vi "RADAR (NI 5791 FPGA).vi"() -> ()   [LabVIEW 2017]
uses:
  <instrlib>/_niInstr/Register Bus/v1/FPGA/Public/Read Cmd Data.ctl
  <instrlib>/_niInstr/DSP/v1/Shared/Public/IQ Gain.ctl
  <instrlib>/_niInstr/DSP/v1/Shared/Public/IQ Impairments.ctl
  <vilib>/Platform/TimedLoop/XDataNode/timing_clust.ctl
  <vilib>/Platform/TimedLoop/XDataNode/nitl_modes.ctl
  <vilib>/Platform/TimedLoop/XDataNode/wakeup.ctl
  <instrlib>/_niInstr/DSP/v1/Shared/Public/IQ Data.ctl
  <instrlib>/ni579x/Synchronization/v2/FPGA/Implementation/Create 5791.vi
  <vilib>/rvi/Emulation/niFpgaSctlEmulationGetInTimedLoop.vi
  <vilib>/rvi/Emulation/niFpgaEmulationReportErrorSimple.vi
  <vilib>/rvi/Emulation/niFpgaGetClockAttributes.vi
  <vilib>/rvi/Emulation/niFpgaCriticalErrorInLSC.vi
  <vilib>/rvi/eio/common/nirviEmuTemplateMethod_errors.vi
  <instrlib>/_niInstr/Register Bus/v1/FPGA/Private/Mux/Read Completion Mux (3 inputs).vi
  <vilib>/rvi/Emulation/niFpgaProcessEmulError.vi
  <instrlib>/_niInstr/DSP/v1/FPGA/Public/Sub VIs/Data Conversion/I16 to IQ - 1 spc - S18.1.vi
  <instrlib>/_niInstr/DSP/v1/FPGA/Public/Sub VIs/Data Conversion/IQ to U32 - 1 spc - S18.1.vi
  <instrlib>/_niInstr/Basic Elements/v1/FPGA/Private/Count Up U64.vi
  <instrlib>/_niInstr/DSP/v1/FPGA/Public/Sub VIs/Data Conversion/U32 to IQ - 1 spc - S18.1.vi
  <instrlib>/_niInstr/DSP/v1/FPGA/Public/Sub VIs/Data Conversion/IQ to I16 - 1 spc - S18.1.vi
  <vilib>/rvi/interface/RandomDataEmulation/niFpgaRandomDataHandleErrors.vi
  <vilib>/rvi/DataTransferAndStorage/Container/Common/niFpgaContainerExecOnDevCompGetState.vi
  <vilib>/rvi/Emulation/niFpgaEmulationIsFPGAContextNoSignature.vi
  <vilib>/rvi/errors/niFpgaSetErrorForExecOnDevCompSimple.vi
  <vilib>/rvi/eio/common/nirviEmuReportErrorAndStop.vi
  <vilib>/rvi/DataTransferAndStorage/Container/Common/niFpgaContainerGetUniqueNameForEmu.vi
  <vilib>/rvi/FIFO/Fifo_Resource/nirvififoEmulationSetSize.vi
  <vilib>/rvi/FIFO/Fifo_Resource/nirviFifoEmulationQueueMgr.vi
  <instcachedir>/0/nirviFifoEmulationQueueMgr_E5CAEC123FF24DC58D834DCA3CDAA9B5.lvgen/nirviFifoEmulationQueueMgr_E5CAEC123FF24DC58D834DCA3CDAA9B5_000.vi
  <vilib>/rvi/FIFO/Fifo_Resource/nirvififoEmulationDetermineInputValidOut.vi
  <vilib>/rvi/FIFO/Fifo_Resource/nirvififoEmulationCreateLock.vi
  <vilib>/rvi/FIFO/Fifo_Resource/nirvififoEmulationObtainLock.vi
  <vilib>/rvi/FIFO/Fifo_Resource/nirvififoEmulationReleaseLock.vi
  <vilib>/rvi/occurrence/nirviWaitOnOccurrenceBase.vi
  <vilib>/rvi/errors/nirviReportUnexpectedCaseInternalError.vi
  <vilib>/rvi/errors/nirviReportUnexpectedCaseInternalError (U32).vi
  <vilib>/Utility/error.llb/Clear Errors.vi
  <instcachedir>/0/nirviFifoEmulationQueueMgr_E5CAEC123FF24DC58D834DCA3CDAA9B5.lvgen/nirviFifoEmulationQueueMgr_E5CAEC123FF24DC58D834DCA3CDAA9B5_003.vi
  <vilib>/Platform/TimedLoop/XDataNode/XDataNode.xnode
  <vilib>/eio/EIONode/EIONode.xnode
  <vilib>/rvi/DataTransferAndStorage/Container/XNode/niFpgaContainer.xnode
  <vilib>/rvi/interface/RandomDataEmulation/nirviRandomDataFpgaReadWriteTemplate.vi
  <vilib>/rvi/FXPMathLib/basic elements/FxpDiscreteDelay/XNode/nifxpmath_DiscreteDelay.xnode
  <vilib>/rvi/FIFO/Fifo_Resource/niFpgaFifoEmulationRefIn.vi
  <vilib>/rvi/FIFO/Fifo_Resource/nirvififoEmulationClear.vi
  <vilib>/Platform/TimedLoop/XDataNode/XDNodeRunTimeDep.lvlib
  <instrlib>/ni579x/Synchronization/v2/FPGA/ni579x Synchronization v2 FPGA.lvlib
  <instrlib>/ni579x/Config/v2/FPGA/ni579x Config v2 FPGA.lvlib
  <instrlib>/_niInstr/Register Bus/v1/FPGA/niInstr Register Bus v1 FPGA.lvlib
  <instrlib>/_niInstr/DSP/v1/FPGA/niInstr DSP v1 FPGA.lvlib
  <instrlib>/_niInstr/DSP/v1/Shared/niInstr DSP v1 Shared.lvlib
  <instrlib>/_niInstr/Basic Elements/v1/FPGA/niInstr Basic Elements v1 FPGA.lvlib
  <vilib>/rvi/Analysis/common/FxpNativeNode/niFpgaFxpNative.xnode
panel:
  out "realimentarTX":u32
  in  "Pulse Energy":fxp<+,32,0>=0.99609375
  out "no_guard":bool
  out "IO Rxy":cluster{i32, i32}(graph)
  out "Rxy I":i32
  out "Rxy Q":i32
  out "Rx after":cluster{"output":i16, "output":i16}(graph)
  out "Rx before":cluster{"f":i16, i16}(graph)
  out "rx.number of IQ data processed":u64
  out "rx.number of IQ data overflows":u64
  out "tx.number of IQ data processed":u64
  out "tx.number of IQ data overflows":u64
  out "IO Rx":cluster{i16, i16}(graph)
  in  "rx.output sample rate":fxp<+,48,1>=1.0
  in  "rx.delay":fxp<+/-,16,0>
  in  "rx.phase":fxp<+/-,21,0> format="%#_4g"
  in  "rx.frequency shift":fxp<+/-,48,0> format="%#.7g"
  in  "rx.impairments":T1={"inline gain I"=0.9999923706054688, "inline gain Q"=0.9999923706054688, "cross gain I"=0.0, "cross gain Q"=0.0, "pre-gain offset I"=0.0, "pre-gain offset Q"=0.0, "post-gain offset I"=0.0, "post-gain offset Q"=0.0} {"post-gain offset Q" format="%#_4g"; "post-gain offset I" format="%#_4g"; "pre-gain offset Q" format="%#_4g"; "pre-gain offset I" format="%#_4g"; "cross gain Q" format="%#_4g"; "cross gain I" format="%#.4g"; "inline gain Q" format="%#.4g"; "inline gain I" format="%#.4g"}
  in  "tx.reset":bool
  in  "rx.reset":bool
  out "Rxy valid":bool
  out "IO Tx":cluster{"I":i16, "Q":i16}(graph)
  in  "tx.impairments":T1={"inline gain I"=0.9999923706054688, "inline gain Q"=0.9999923706054688, "cross gain I"=0.0, "cross gain Q"=0.0, "pre-gain offset I"=0.0, "pre-gain offset Q"=0.0, "post-gain offset I"=0.0, "post-gain offset Q"=0.0} {"post-gain offset Q" format="%#_4g"; "post-gain offset I" format="%#_4g"; "pre-gain offset Q" format="%#_4g"; "pre-gain offset I" format="%#_4g"; "cross gain Q" format="%#_4g"; "cross gain I" format="%#.4g"; "inline gain Q" format="%#_4g"; "inline gain I" format="%#_4g"}
  in  "tx.phase":fxp<+/-,21,0> format="%#_4g"
  in  "tx.frequency shift":fxp<+/-,48,0> format="%#.4g"
  in  "tx.delay":fxp<+/-,18,0>
  in  "tx.input sample rate":fxp<+,48,1>
  in  "tx.gain":T2={"gain I"=1.0, "gain Q"=1.0}
  in  "Chip width":u16
  in  "sign":bool
  in  "Beta/tao":fxp<+,52,48>=7000000000000.0
  in  "Beta":fxp<+,26,24>=7000000.0 format="%#.3p"
  in  "N":u8=1
  in  "Delta":u8=130
  in  "Guard width":u16=130
  in  "Oversampling factor":u8=1
  in  "Select Wave":u8
  out "start_Rx":bool
  out "end_Rx":bool
  out "end_Tx":bool
  out "start_Tx":bool
  in  "Pulse width":u16=130
  in  "PRP":u32=1300 caption="(in ticks of 130MHz)"
  out "Generation":cluster{"cte I":i16, "cte Q":i16}(graph)
  in  "cte Q":i16
  in  "cte I":i16=16384
  in  "reg.host read.go rcvd 0":bool
  out "reg.notify host.go 0":bool
  in  "reg.notify host.go rcvd 0":bool
  out "reg.host read.data 0":T3
  in  "reg.reset 0":bool
  out "IO Module\\Initialization Done":bool
  out "IO Module\\PLL Locked":bool
  out "IO Module\\LO Locked":bool
  out "IO Module\\User Error":u8
  # "Radar Parameters"
  # "REGISTER BUS"
  # "(in ticks of 130MHz)"
  # "* Calculated on host side"
  # "*"
  # "*"
  # "Case 0: constants (I/Q)\nCase 1: Chirp (I/Q) Generation Panel \nCase 2: Barker 7 code (I: +1,+1,+1,-1,-1,+1,-1 / Q: 0)\nCase 3: Barker 13 code (I: +1,+1,+1,+1,+1,-1,-1,+1,+1,-1,+1,-1,+1 / Q: 0)"
  # "Required Controls & Indicators"
  # "Constant Wave Generation"
  # "Chirp Wave Generation"
  # "Barker Wave Generation"
  # "*"
  # "*"
  # "Tx Signal Conditioner & Stats"
  # "Rx Signal Conditioner & Stats"
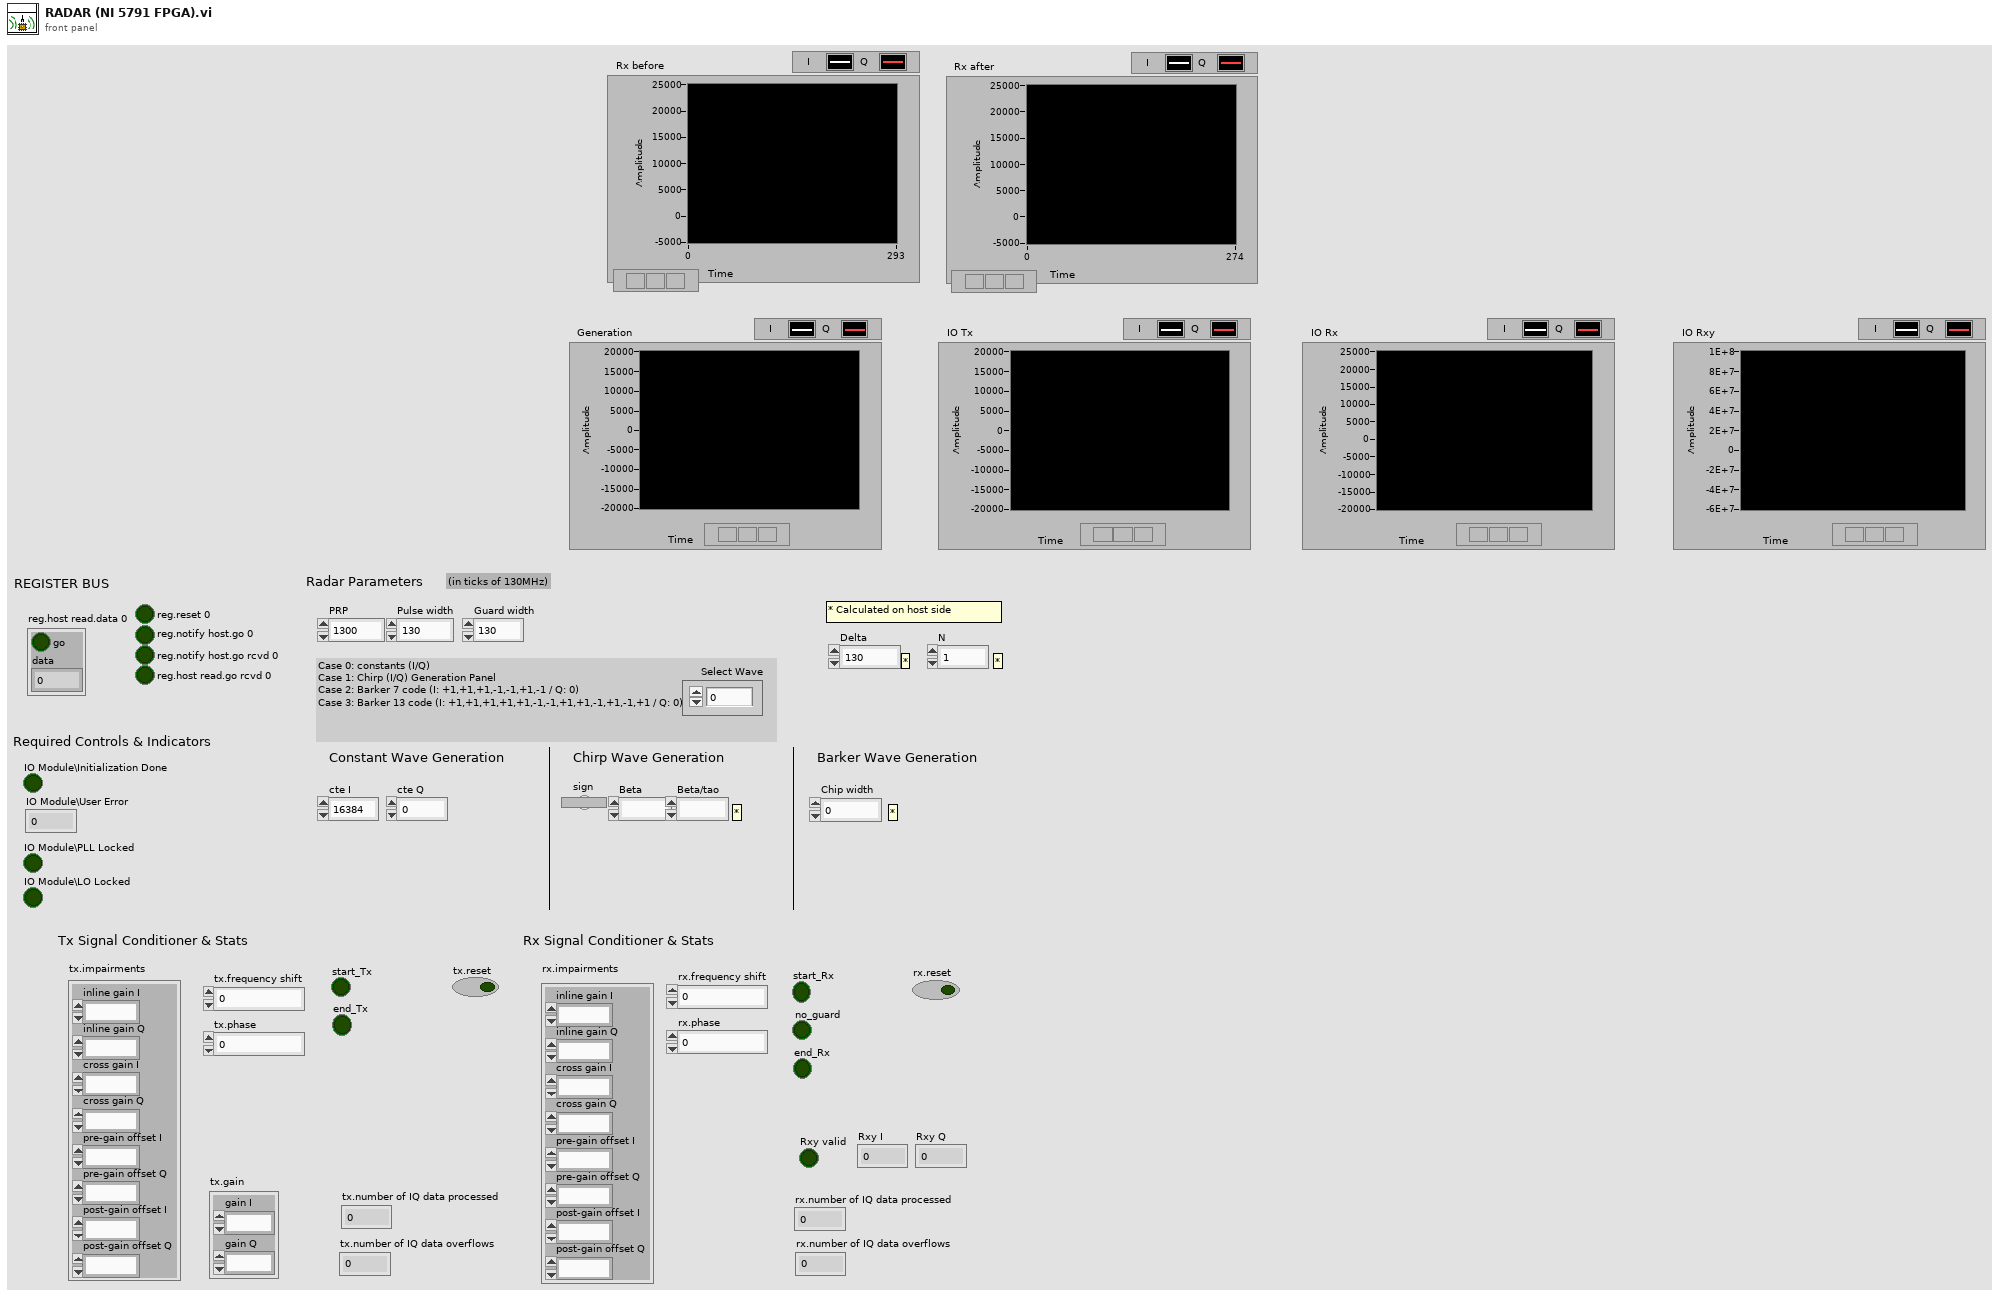
[diagram p1: front panel]
types:
  T1 = typedef "niInstr DSP v1 Shared.lvlib/IQ Impairments.ctl" = cluster{"inline gain I":fxp<+/-,18,1>, "inline gain Q":fxp<+/-,18,1>, "cross gain I":fxp<+/-,18,1>, "cross gain Q":fxp<+/-,18,1>, "pre-gain offset I":fxp<+/-,18,1>, "pre-gain offset Q":fxp<+/-,18,1>, "post-gain offset I":fxp<+/-,18,1>, "post-gain offset Q":fxp<+/-,18,1>}
  T2 = typedef "niInstr DSP v1 Shared.lvlib/IQ Gain.ctl" = cluster{"gain I":fxp<+/-,24,3>, "gain Q":fxp<+/-,24,3>}
  T3 = typedef "niInstr Register Bus v1 FPGA.lvlib/Read Cmd Data.ctl" = cluster{"go":bool, "data":u32}
  T4 = typedef "XDNodeRunTimeDep.lvlib/timing_clust.ctl" = cluster{"Expected End [f-1]":u64, "Actual End [f-1]":u64, "Finished Late? [f-1]":bool, "Expected End [i-1]":u64, "Actual End [i-1]":u64, "Finished Late? [i-1]":bool, "Expected Start [i]":u64, "Actual Start [i]":u64, "Expected Start [f]":u64, "Actual Start [f]":u64, "Source Name":string, "Structure Name":string, "Period":i64, "Deadline":i64, "Offset":i64, "Start":i64, "Priority":i32, "Timeout":i32, "Mode":T5, "Wakeup Reason":T6, "Error":errorcluster, "Source Type":string, "Secondary Source Type":string, "Global End Time":u64, "Global Start Time":u64, "Frame Duration":u64, "Iteration Duration":u64, "Assigned CPU":i32, "I/O Scan Engine Mode":u32}
  T5 = typedef "XDNodeRunTimeDep.lvlib/nitl_modes.ctl" = enum32{"No Change", "Process missed periods, maintain original phase", "Discard missed periods, maintain original phase", "Process missed periods, ignore original phase", "Discard missed periods, ignore original phase"}
  T6 = typedef "XDNodeRunTimeDep.lvlib/wakeup.ctl" = enum32{"Normal", "Aborted", "Asynchronous wakeup", "Timing source error", "Timed loop error", "Timeout"}
  T7 = typedef "ni579x Synchronization v2 FPGA.lvlib/Resources.ctl" = cluster{"master":refnum<k21>, "meas.enable":refnum<k21>, "meas.ready":refnum<k21>, "meas.arm":refnum<k21>, "meas.valid":refnum<k21>, "meas.value":refnum<k21>, "meas.oversample clock":refnum<k21>, "meas.oversample factor":refnum<k21>, "cptr":refnum<k21>, "cptr.adjust":refnum<k21>, "cptr.period":refnum<k21>}
  T8 = typedef "niInstr Register Bus v1 FPGA.lvlib/Register Instruction.ctl" = cluster{"subsystem":u8, "address":u16, "data":u32, "valid":bool, "read":bool}
  T9 = typedef "niInstr Register Bus v1 FPGA.lvlib/Read Completion.ctl" = cluster{"data":u32, "valid":bool}
  T10 = typedef "niInstr DSP v1 Shared.lvlib/IQ Data.ctl" = cluster{"I":fxp<+/-,18,1>, "Q":fxp<+/-,18,1>, "overflow":bool}
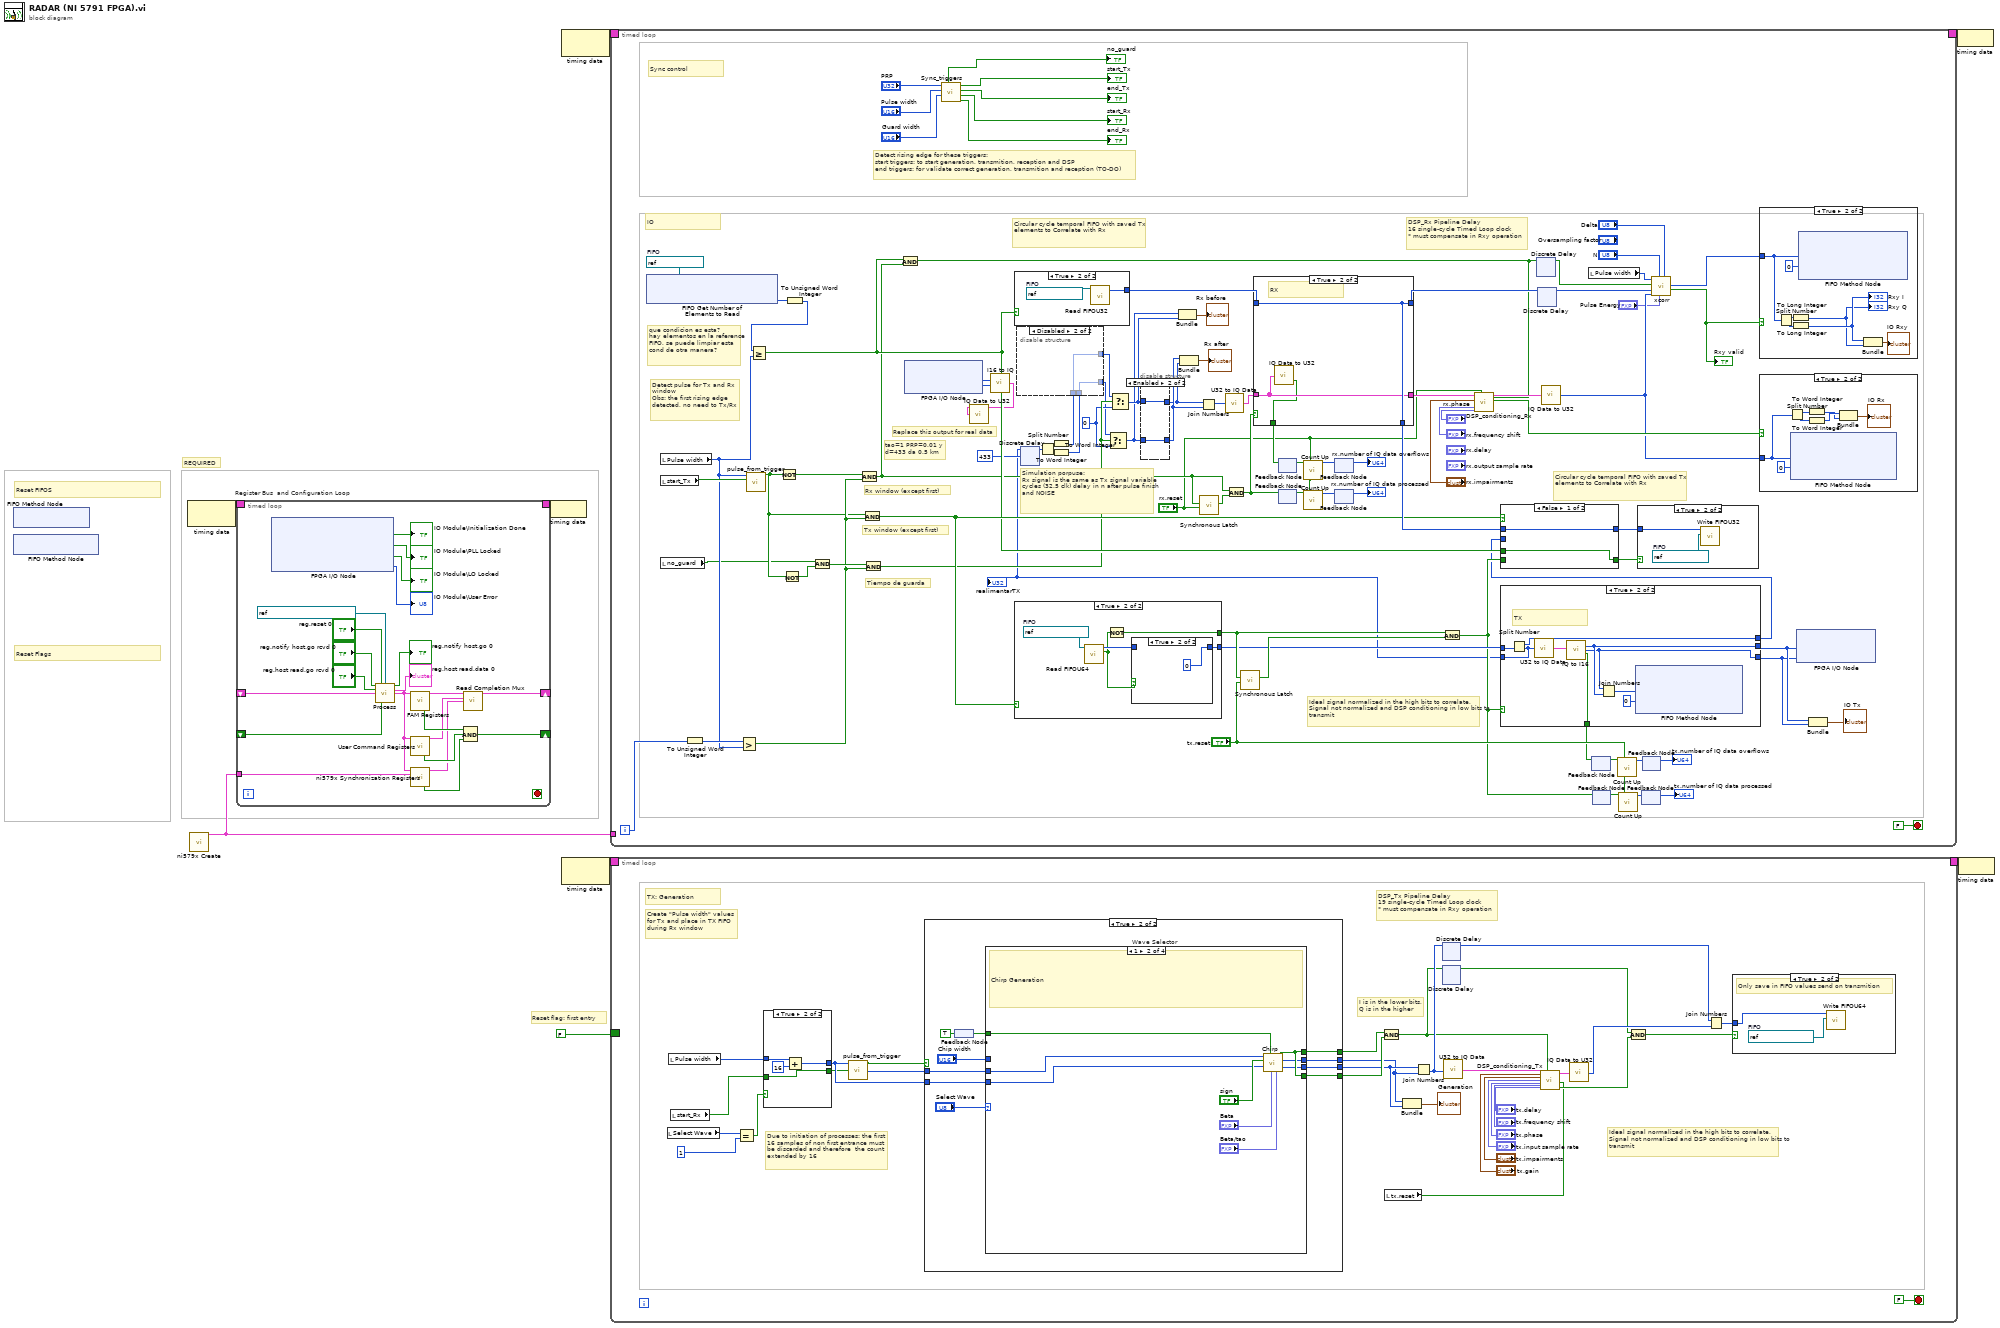
[diagram p0: block diagram]
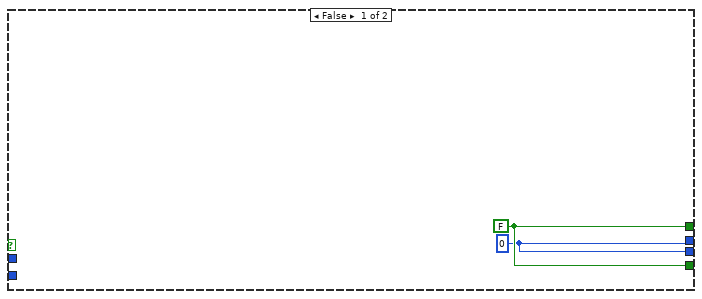
[diagram p3: hidden frame]
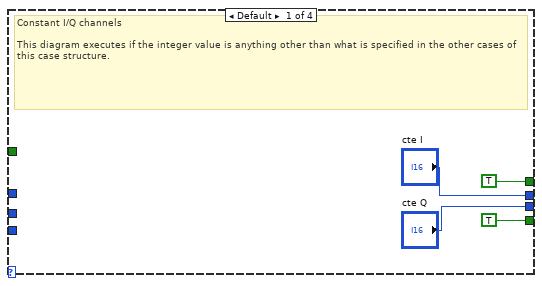
[diagram p4: hidden frame]
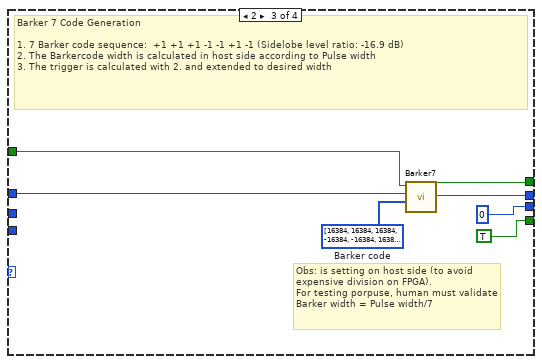
[diagram p5: hidden frame]
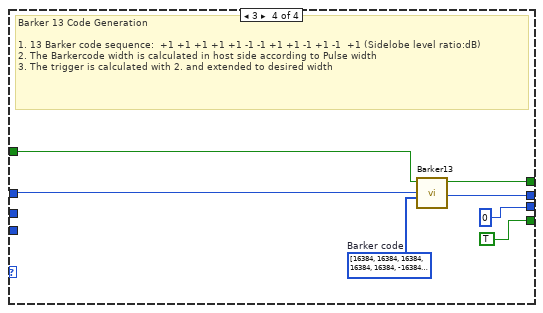
[diagram p6: hidden frame]
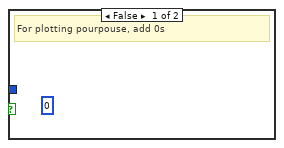
[diagram p7: hidden frame]
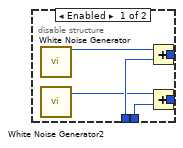
[diagram p8: hidden frame]
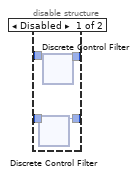
[diagram p10: hidden frame]
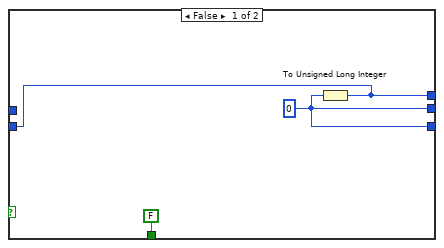
[diagram p12: hidden frame]
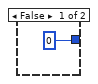
[diagram p13: hidden frame]
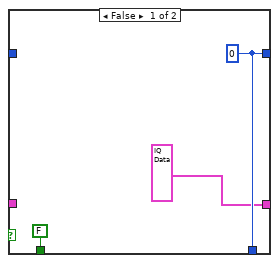
[diagram p16: hidden frame]
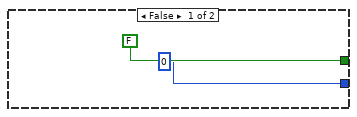
[diagram p17: hidden frame]
diagram:
  # "Reset Flags"
  # "Reset FIFOS"
  # "Reset flag: first entry"
  # "REQUIRED"
  n1 = xnode ("FIFO Method Node")() -> ()  [unwired: 1 in, 1 out]
  n2 = xnode ("FIFO Method Node")() -> ()  [unwired: 1 in, 1 out]
  n3 = node-c288() -> (w8:T4)  [unwired: 1 in]
  n4 = call-poly <instrlib>:"ni579x Create.vi"() -> ("sync.resources"=w6:T7)  [unwired: 15 in]
  n5 = timed-loop "Register Bus  and Configuration Loop" {
    timing: w8 -> [_]
    timing-out: [_] -> w7
    shift-right: [w23] -> _
    shift-left: _ -> [w22]
    shift-right: [w21] -> _
    shift-left: _ -> [w20]
    tunnel: w6 -> [w9]
    stop <- _ stop-if-true
    n6 = xnode "FPGA I/O Node"() -> ("IO Module\\Initialization Done"=→"IO Module\\Initialization Done":bool, "IO Module\\PLL Locked"=→"IO Module\\PLL Locked":bool, "IO Module\\LO Locked"=→"IO Module\\LO Locked":bool, "IO Module\\User Error"=→"IO Module\\User Error":u8)  [unwired: 4 in, 4 out]
    n7 = call <instrlib>:"Process.vi"("reg.notify host.go rcvd"="reg.notify host.go rcvd 0", "reg.reset"="reg.reset 0", "reg.host instruction fifo"=refnum<k21> "reg.host instruction fifo 0", "reg.host read.go rcvd"="reg.host read.go rcvd 0", "read completion"=w22, "ready for output"=w20) -> ("reg.notify host.go"=→"reg.notify host.go 0":bool, "reg.host read.data"=→"reg.host read.data 0":T3, "register instruction"=w12:T8)  [unwired: 7 in]
    n8 = call <instrlib>:"FAM Registers.vi"("register instruction"=w12) -> ("read completion"=w25:T9, "ready for input"=w27:bool)  [unwired: 12 in, 1 out]
    n9 = call <instrlib>:"User Command Registers.vi"("register instruction"=w12) -> ("read completion"=w24:T9, "ready for input"=w26:bool)  [unwired: 11 in, 2 out]
    n10 = call <instrlib>:"ni579x Synchronization Registers.vi"("register instruction"=w12, "sync.resources"=w9) -> ("read completion"=w11:T9, "ready for input"=w10:bool)  [unwired: 12 in]
    n11 = call-poly <instrlib>:"Read Completion Mux.vi"("element 0"=w25, "element 1"=w24, "element 2"=w11) -> ("read completion out"=w23:T9)  [unwired: 12 in]
    n12 = Compound Arithmetic op=AND(w27, w26, w10) -> (w21:bool)
  }
  n13 = node-c288(w7) -> ()
  n14 = node-c288() -> (w5:T4)  [unwired: 1 in]
  n15 = node-c288() -> (w3:T4)  [unwired: 1 in]
  n16 = timed-loop {
    timing: w5 -> [_]
    timing-out: [_] -> w4
    tunnel: w6 -> [_]
    i -> [w58]
    stop <- FALSE stop-if-true
    w65 = i16 0 ("f")
    w115 = refnum<k21> "Tx reference"  # FIFO
    # "tao=1 PRP=0.01 y \nd=433 da 0.5 km"
    # "Ideal signal normalized in the high bits to correlate,\nSignal not normalized and DSP conditioning in low bits to transmit"
    # "Circular cycle temporal FIFO with saved Tx elements to Correlate with Rx"
    # "que condicion es esta?\nhay elementos en la reference FIFO, se puede limpiar esta cond de otra manera?"
    # "Rx window (except first)"
    # "Tx window (except first)"
    # "DSP_Rx Pipeline Delay \n16 single-cycle Timed Loop clock \n* must compensate in Rxy operation"
    # "Replace this output for real data"
    # "Circular cycle temporal FIFO with saved Tx elements to Correlate with Rx"
    # "Detect pulse for Tx and Rx window\nObs: the first rising edge detected, no need to Tx/Rx"
    # "Simulation porpuse:\nRx signal is the same as Tx signal variable cycles (32.5 clk) delay in n after pulse finish and NOISE"
    # "Tiempo de guarda"
    # "IO"
    # "Detect rising edge for these triggers:\nstart triggers: to start generation, transmition, reception and DSP\nend triggers: for validate correct generation, transmition and reception (TO-DO)"
    # "Sync control"
    n17 = xnode ("FIFO Get Number of Elements to Read")("FIFO In"=w115) -> ("Number of Elements to Read"=w35:u32)  [unwired: 1 out]
    n18 = local read "Pulse width"() -> (w49:u16)
    n19 = local read "start_Tx"() -> (w50:bool)
    n20 = local read "no_guard"() -> (w39:bool)
    n21 = To Unsigned Word Integer(number=w58) -> (unsigned 16bit integer=w108:u16)
    n22 = Greater?(x=w108, y=w49) -> (0:w63:bool)
    n23 = call "pulse_from_trigger.vi"("trigger"=w50, "Pulse width"=w49) -> ("pulse"=w41:bool)  [unwired: 8 in, 1 out]
    n24 = Not(x=w41) -> (.not. x?=w69:bool)
    n25 = Not(x=w41) -> (.not. x?=w70:bool)
    n26 = To Unsigned Word Integer(number=w35) -> (unsigned 16bit integer=w34:u16)
    n27 = Greater Or Equal?(x=w34, y=w49) -> (x >= y?=w113:bool)
    n28 = And(x=w39, y=w70) -> (x .and. y?=w64:bool)
    n29 = And(x=w69, y=w63) -> (x .and. y?=w62:bool)
    n30 = And(x=w41, y=w63) -> (x .and. y?=w114:bool)
    n31 = And(x=w64, y=w63) -> (x .and. y?=w68:bool)
    n32 = And(x=w113, y=w62) -> (x .and. y?=w98:bool)
    n33 = xnode "FPGA I/O Node"() -> ("IO Module\\Rx I"=w97:i16, "IO Module\\Rx Q"=w96:i16)  [unwired: 2 in, 2 out]
    n34 = call "Sync_triggers.vi"("PRP"="PRP", "Pulse width"="Pulse width", "Guard width"="Guard width") -> ("no_guard"=→"no_guard":bool, "end_Rx"=→"end_Rx":bool, "start_Tx"=→"start_Tx":bool, "end_Tx"=→"end_Tx":bool, "start_Rx"=→"start_Rx":bool)  [unwired: 1 in]
    n35 = call-poly <instrlib>:"I16 to IQ.vi"("I"=w97, "Q"=w96) -> ("IQ"=w60:T10)  [unwired: 13 in]
    n36 = call-poly <instrlib>:"IQ Data to U32.vi"("IQ data"=w60) -> ()  [unwired: 13 in, 2 out]
    n37 = case shown="True" w113 {
      tunnel: [u32 0 ("Element") w230] -> w110
      frame False {
      }
      frame True {
        w231 = refnum<k21> "Tx reference"  # FIFO
        n38 = call "Read FIFOU32.vi"("Refnum in"=w231) -> ("Element"=w230:u32)  [unwired: 9 in, 1 out]
      }
    }
    n39 = case shown="True" w114 {
      tunnel: [u32 0 ("Element") w248] -> w105
      tunnel: [FALSE ("Timed Out?") w247] -> w107
      frame False {
      }
      frame True {
        w249 = refnum<k21> "Tx Signal FPGA"  # FIFO
        n40 = call "Read FIFOU64.vi"("Refnum in"=w249) -> ("Timed Out?"=w246:bool, "Element"=w250:u64)  [unwired: 9 in]
        n41 = Not(x=w246) -> (.not. x?=w247:bool)
        n42 = case shown="True" w246 {
          tunnel: w250 -> [w251 _]
          tunnel: [w251 u64 0 ("Element")] -> w248
          frame False {
            # "Save Tx for Rxy"
          }
          frame True {
          }
        }
      }
    }
    n43 = call <instrlib>:"Synchronous Latch.vi"("clear"="rx.reset", "set"=w62) -> ("out"=w61:bool)  [unwired: 9 in]
    n44 = And(x=w62, y=w61) -> (x .and. y?=w43:bool)
    n45 = call <instrlib>:"Synchronous Latch.vi"("clear"="tx.reset", "set"=w107) -> ("out"=w106:bool)  [unwired: 9 in]
    n46 = feedback #1() -> (w85:bool)  [unwired: 1 in]
    n47 = feedback #2() -> (w81:bool)  [unwired: 1 in]
    n48 = feedback-in #2(w43) -> ()
    n49 = call-poly <instrlib>:"Count Up.vi"("increment"=w85, "reset"="rx.reset") -> ("count out"=w87:u64)  [unwired: 13 in]
    n50 = call-poly <instrlib>:"Count Up.vi"("increment"=w81, "reset"="rx.reset") -> ("count out"=w84:u64)  [unwired: 13 in]
    n51 = feedback #3() -> (→"rx.number of IQ data overflows":u64)  [unwired: 1 in]
    n52 = feedback-in #3(w87) -> ()
    n53 = feedback #4() -> (→"rx.number of IQ data processed":u64)  [unwired: 1 in]
    n54 = feedback-in #4(w84) -> ()
    n55 = And(x=w107, y=w106) -> (x .and. y?=w73:bool)
    n56 = case shown="True" w73 {
      tunnel: [w218 w226] -> w112
      tunnel: [w218 w222] -> w111
      tunnel: w105 -> [_ w224]
      tunnel: [w217 w223] -> w59
      tunnel: [FALSE ("overflow") w221] -> w88
      tunnel: [w217 w220] -> w33
      frame False {
        w218 = i16 0 ("Q")
        n57 = To Unsigned Long Integer(number=w218) -> (unsigned 32bit integer=w217:u32)
      }
      frame True {
        # "TX"
        n58 = Split Number(x=w224) -> (hi(x)=w223:u32, lo(x)=w220:u32)
        n59 = call-poly <instrlib>:"U32 to IQ Data.vi"("U32 data"=w220) -> ("IQ data"=w225:T10)  [unwired: 14 in]
        n60 = call-poly <instrlib>:"IQ to I16.vi"("IQ"=w225) -> ("I"=w226:i16, "Q"=w222:i16, "overflow"=w221:bool)  [unwired: 12 in]
        n61 = Join Numbers(hi=w222, lo=w226) -> ((hi.lo)=w227:u32)
        n62 = xnode ("FIFO Method Node")("Element"=w227, "Timeout"=0) -> ()  [unwired: 1 in, 2 out]
      }
    }
    "realimentarTX" <- w33
    n63 = xnode ("Discrete Delay")("D"=w33, "n-1[0..511]"=u16 433) -> ("Q"=w77:u32)
    n64 = Split Number(x=w77) -> (hi(x)=w76:u16, lo(x)=w75:u16)
    n65 = To Word Integer(number=w76) -> (16bit integer=w47:i16)
    n66 = To Word Integer(number=w75) -> (16bit integer=w46:i16)
    n67 = disable-structure shown="Disabled" {
      disable-tunnel: w47 -> [w132 w134]
      disable-tunnel: w46 -> [w131 w133]
      disable-tunnel: [w130 w134] -> w45
      disable-tunnel: [w129 w133] -> w44
      frame Enabled {
        n68 = call "White Noise Generator"() -> ("white noise out"=w128:i16)  [unwired: 15 in]
        n69 = call "White Noise Generator2"() -> ("white noise out"=w127:i16)  [unwired: 15 in]
        n70 = Add(x=w128, y=w132) -> (x+y=w130:i16)
        n71 = Add(x=w127, y=w131) -> (x+y=w129:i16)
      }
      frame Disabled {
      }
    }
    n72 = Select(t=w44, s=w68, f=w65) -> (s? t:f=w66:i16)
    n73 = Select(t=w45, s=w68, f=w65) -> (s? t:f=w67:i16)
    n74 = disable-structure shown="Enabled" {
      disable-tunnel: [w145 w208] -> w72
      disable-tunnel: [w144 w209] -> w71
      disable-tunnel: w67 -> [w143 w209]
      disable-tunnel: w66 -> [w142 w208]
      frame Disabled {
        n75 = xnode "Discrete Control Filter"("input"=w142) -> ("output"=w145:i16)  [unwired: 1 in]
        n76 = xnode "Discrete Control Filter"("input"=w143) -> ("output"=w144:i16)  [unwired: 1 in]
      }
      frame Enabled {
      }
    }
    n77 = Bundle("f"=w66, "f"=w67) -> (→"Rx before":cluster{"f":i16, "f":i16})  [unwired: 1 in]
    n78 = Bundle("f"=w72, "f"=w71) -> (→"Rx after":cluster{"f":i16, "f":i16})  [unwired: 1 in]
    n79 = Join Numbers(hi=w71, lo=w72) -> ((hi.lo)=w78:u32)
    n80 = call-poly <instrlib>:"U32 to IQ Data.vi"("U32 data"=w78) -> ("IQ data"=w74:T10)  [unwired: 14 in]
    n81 = case shown="True" w43 {
      tunnel: [w239 w243] -> w118
      tunnel: w110 -> [_ w243]
      tunnel: [w239 w243] -> w109
      tunnel: w74 -> [_ w242]
      tunnel: [T10 {"I"=0.0, "Q"=0.0, "overflow"=FALSE} ("IQ data") w242] -> w101
      tunnel: [FALSE ("overflow") w241] -> w82
      frame False {
        w239 = u32 0 ("Q")
      }
      frame True {
        # "RX"
        n82 = call-poly <instrlib>:"IQ Data to U32.vi"("IQ data"=w242) -> ("overflow"=w241:bool)  [unwired: 13 in, 1 out]
      }
    }
    n83 = feedback-in #1(w82) -> ()
    n84 = call "DSP_conditioning_Rx.vi"("rx.input valid"=w98, "rx.frequency shift"="rx.frequency shift", "rx.reset"="rx.reset", "rx.phase"="rx.phase", "rx.impairments"="rx.impairments", "data in"=w101) -> ("output valid"=w99:bool, "data out"=w100:T10)  [unwired: 3 in, 1 out]
    n85 = case shown="False" w114 {
      tunnel: w59 -> [_ w237]
      tunnel: w118 -> [w235 _]
      tunnel: [w235 w237] -> w116
      tunnel: w73 -> [_ w236]
      tunnel: [w234 w236] -> w117
      tunnel: w113 -> [w234 _]
      frame False {
      }
      frame True {
      }
    }
    n86 = xnode ("Discrete Delay")("D"=w98) -> ("Q"=w54:bool)
    n87 = xnode ("Discrete Delay")("D"=w109) -> ("Q"=w55:u32)
    n88 = call-poly <instrlib>:"IQ Data to U32.vi"("IQ data"=w100) -> ("U32 data"=w56:u32)  [unwired: 13 in, 1 out]
    n89 = local read "Pulse width"() -> (w57:u16)
    n90 = feedback #5() -> (w94:bool)  [unwired: 1 in]
    n91 = feedback-in #5(w88) -> ()
    n92 = feedback #6() -> (w90:bool)  [unwired: 1 in]
    n93 = feedback-in #6(w73) -> ()
    n94 = call-poly <instrlib>:"Count Up.vi"("increment"=w94, "reset"="tx.reset") -> ("count out"=w95:u64)  [unwired: 13 in]
    n95 = call-poly <instrlib>:"Count Up.vi"("increment"=w90, "reset"="tx.reset") -> ("count out"=w92:u64)  [unwired: 13 in]
    n96 = case shown="True" w117 {
      tunnel: w116 -> [_ w232]
      frame False {
      }
      frame True {
        w233 = refnum<k21> "Tx reference"  # FIFO
        n97 = call "Write FIFOU32.vi"("FIFO In"=w233, "Numeric"=w232) -> ()  [unwired: 10 in]
      }
    }
    n98 = feedback #7() -> (→"tx.number of IQ data processed":u64)  [unwired: 1 in]
    n99 = feedback-in #7(w92) -> ()
    n100 = feedback #8() -> (→"tx.number of IQ data overflows":u64)  [unwired: 1 in]
    n101 = feedback-in #8(w95) -> ()
    n102 = call "xcorr.vi"("Delta"="Delta", "Pulse Energy"="Pulse Energy", "N"="N", "y"=w56, "x"=w55, "enable"=w54, "tao"=w57) -> ("Rxy valid"=w52:bool, "Rxy"=w53:u64)  [unwired: 1 in, 1 out]
    "Rxy valid" <- w52
    n103 = case shown="True" w52 {
      tunnel: w53 -> [_ w138]
      frame False {
      }
      frame True {
        n104 = Split Number(x=w138) -> (hi(x)=w140:u32, lo(x)=w139:u32)
        n105 = To Long Integer(number=w140) -> (32bit integer=w135:i32)
        "Rxy Q" <- w135
        n106 = To Long Integer(number=w139) -> (32bit integer=w136:i32)
        "Rxy I" <- w136
        n107 = xnode ("FIFO Method Node")("Element"=w138, "Timeout"=0) -> ()  [unwired: 1 in, 2 out]
        n108 = Bundle(w136, w135) -> (→"IO Rxy":cluster{i32, i32})  [unwired: 1 in]
      }
    }
    n109 = case shown="True" w99 {
      tunnel: w56 -> [_ w210]
      frame False {
      }
      frame True {
        n110 = Split Number(x=w210) -> (hi(x)=w216:u16, lo(x)=w214:u16)
        n111 = xnode ("FIFO Method Node")("Element"=w210, "Timeout"=0) -> ()  [unwired: 1 in, 2 out]
        n112 = To Word Integer(number=w216) -> (16bit integer=w212:i16)
        n113 = To Word Integer(number=w214) -> (16bit integer=w213:i16)
        n114 = Bundle(w213, w212) -> (→"IO Rx":cluster{i16, i16})  [unwired: 1 in]
      }
    }
    n115 = xnode "FPGA I/O Node"("IO Module\\Tx I"=w112, "IO Module\\Tx Q"=w111) -> ()  [unwired: 2 in, 2 out]
    n116 = Bundle("I"=w112, "Q"=w111) -> (→"IO Tx":cluster{"I":i16, "Q":i16})  [unwired: 1 in]
  }
  n117 = timed-loop {
    timing: w3 -> [_]
    timing-out: [_] -> w2
    border: FALSE -> [_]
    stop <- FALSE stop-if-true
    # "Ideal signal normalized in the high bits to correlate,\nSignal not normalized and DSP conditioning in low bits to transmit"
    # "DSP_Tx Pipeline Delay \n19 single-cycle Timed Loop clock \n* must compensate in Rxy operation"
    # "I is in the lower bits,\nQ is in the higher"
    # "Due to initiation of processes: the first 16 samples of non first entrance must be discarded and therefore  the count extended by 16"
    # "TX: Generation"
    # "Create \"Pulse width\" values for Tx and place in TX FIFO during Rx window"
    n118 = local read "Select Wave"() -> (w281:u8)
    n119 = local read "Pulse width"() -> (w285:u16)
    n120 = local read "start_Rx"() -> (w284:bool)
    n121 = Equal?(x=w281, y=u8 1) -> (x = y?=w283:bool)
    n122 = case shown="True" w283 {
      tunnel: w284 -> [w287 w292]
      tunnel: w285 -> [w288 w291]
      tunnel: [w288 w290] -> w259
      tunnel: [w287 w292] -> w258
      frame False {
      }
      frame True {
        n123 = Add(x=w291, y=u16 16 ("x")) -> (x+y=w290:u16)
      }
    }
    n124 = call "pulse_from_trigger.vi"("trigger"=w258, "Pulse width"=w259) -> ("count"=w260:u16, "pulse"=w257:bool)  [unwired: 8 in]
    n125 = case shown="True" w257 {
      tunnel: [w293 w303] -> w266
      tunnel: [w293 w302] -> w265
      tunnel: [w294 w301] -> w267
      tunnel: [w294 w300] -> w264
      tunnel: w260 -> [_ w295]
      tunnel: w259 -> [_ w296]
      frame False {
        w293 = i16 0 ("cte I")
        w294 = FALSE ("output valid")
      }
      frame True {
        n126 = feedback #9() -> (w298:bool)
        n127 = feedback-in #9(TRUE) -> ()
        n128 = case "Wave Selector" shown="1" "Select Wave" {
          tunnel: ["cte Q" w315 i16 0 ("number: 0 to 6") i16 0 ("number: 0 to 6")] -> w303
          tunnel: ["cte I" w316 w323 w327] -> w302
          tunnel: [TRUE ("output valid") w317 w324 w328] -> w300
          tunnel: [TRUE ("output valid") w317 TRUE ("output valid") TRUE ("output valid")] -> w301
          tunnel: w298 -> [_ w314 w322 w330]
          tunnel: "Chip width" -> [_ _ w318 w329]
          tunnel: w296 -> [_ w311 _ _]
          tunnel: w295 -> [_ w310 _ _]
          frame Default {
            # "Constant I/Q channels \n\nThis diagram executes if the integer value is anything other than what is specified in the other cases of this case structure."
          }
          frame 1 {
            # "Chirp Generation"
            n129 = call "Chirp.vi"("Beta/tao"="Beta/tao", "Beta"="Beta", "first?"=w314, "Pulse width"=w311, "sign"="sign", "count"=w310) -> ("Q"=w315:i16, "I"=w316:i16, "output valid"=w317:bool)  [unwired: 3 in]
          }
          frame 2 {
            w319 = i16[] [16384, 16384, 16384, -16384, -16384, 16384, -16384]  # Barker code
            # "Obs: is setting on host side (to avoid expensive division on FPGA).\nFor testing porpuse, human must validate Barker width = Pulse width/7"
            # "Barker 7 Code Generation\n\n1. 7 Barker code sequence: \t+1 +1 +1 -1 -1 +1 -1\t(Sidelobe level ratio: -16.9 dB)\n2. The Barkercode width is calculated in host side according to Pulse width \n3. The trigger is calculated with 2. and extended to desired width"
            n130 = call "Barker7.vi"("Barker code"=w319, "Barker width"=w318, "first?"=w322) -> ("output"=w323:i16, "output valid"=w324:bool)  [unwired: 7 in]
          }
          frame 3 {
            w331 = i16[] [16384, 16384, 16384, 16384, 16384, -16384, -16384, 16384, 16384, -16384, 16384, -16384, 16384]  # Barker code
            # "Barker 13 Code Generation\n\n1. 13 Barker code sequence: \t+1 +1 +1 +1 +1 -1 -1 +1 +1 -1 +1 -1 \t+1 (Sidelobe level ratio:dB)\n2. The Barkercode width is calculated in host side according to Pulse width \n3. The trigger is calculated with 2. and extended to desired width"
            n131 = call "Barker13.vi"("Barker code"=w331, "Chip width"=w329, "first?"=w330) -> ("output"=w327:i16, "output valid"=w328:bool)  [unwired: 7 in]
          }
        }
      }
    }
    n132 = And(x=w264, y=w267) -> (x .and. y?=w269:bool)
    n133 = local read "tx.reset"() -> (w255:bool)
    n134 = Bundle("output"=w265, "number: 0 to 6"=w266) -> (→"Generation":cluster{"output":i16, "number: 0 to 6":i16})  [unwired: 1 in]
    n135 = Join Numbers(hi=w266, lo=w265) -> ((hi.lo)=w271:u32)
    n136 = xnode ("Discrete Delay")("D"=w271) -> ("Q"=w268:u32)
    n137 = xnode ("Discrete Delay")("D"=w269) -> ("Q"=w270:bool)
    n138 = call-poly <instrlib>:"U32 to IQ Data.vi"("U32 data"=w271) -> ("IQ data"=w274:T10)  [unwired: 14 in]
    n139 = call "DSP_conditioning_Tx.vi"("reset"=w255, "tx.frequency shift"="tx.frequency shift", "IQ data"=w274, "tx.phase"="tx.phase", "input valid"=w269, "tx.delay"="tx.delay", "tx.impairments"="tx.impairments", "tx.input sample rate"="tx.input sample rate", "tx.gain"="tx.gain") -> ("tx.dsp reset done"=w256:bool, "data out"=w273:T10)  [unwired: 1 out]
    n140 = call-poly <instrlib>:"IQ Data to U32.vi"("IQ data"=w273) -> ("U32 data"=w272:u32)  [unwired: 13 in, 1 out]
    n141 = And(x=w270, y=w256) -> (x .and. y?=w263:bool)
    n142 = Join Numbers(hi=w268, lo=w272) -> ((hi.lo)=w262:u64)
    n143 = case shown="True" w263 {
      tunnel: w262 -> [_ w332]
      frame False {
        (unwired) i16 0 ("cte I")
        # "For plotting pourpouse, add 0s"
      }
      frame True {
        w333 = refnum<k21> "Tx Signal FPGA"  # FIFO
        # "Only save in FIFO values send on transmition"
        n144 = call "Write FIFOU64.vi"("FIFO In"=w333, "Numeric"=w332) -> ()  [unwired: 10 in]
      }
    }
  }
  n145 = node-c288(w4) -> ()
  n146 = node-c288(w2) -> ()
